vi "add scan PZT at temp.vi"(10 "字符串":string) -> (1 "ok or cancel":bool, 2 "连接的字符串":string)   [LabVIEW 2019, in "nematic.lvlib"]
uses:
  nematic.lvlib
panel:
  out "数组 2":i32[](array[numeric])
  out "布尔":bool
  in  "最大电压":dbl=148.0
  in  "最小电压":dbl=-48.0
  in  "ok 2":bool
  in  "cancel":bool
  in  "ok":bool
  in  "零电压":dbl
  in  "间隔":dbl=4.0
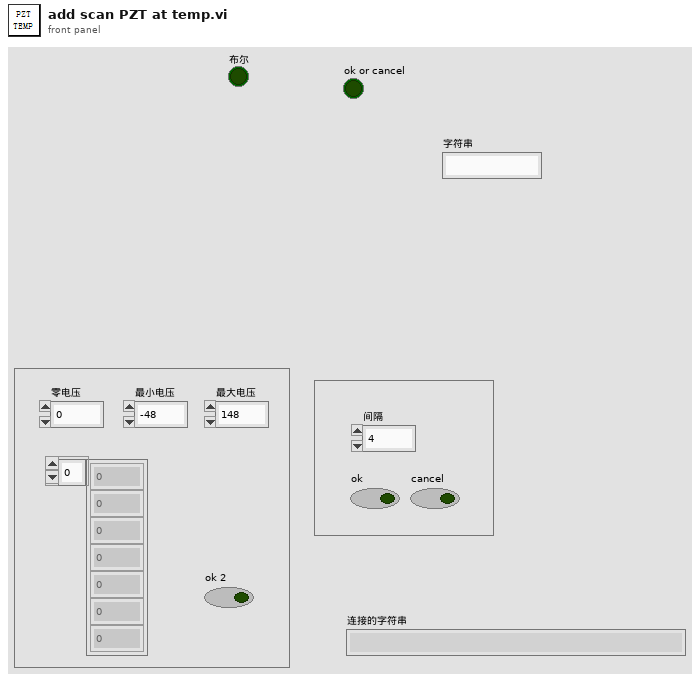
[diagram p1: front panel]
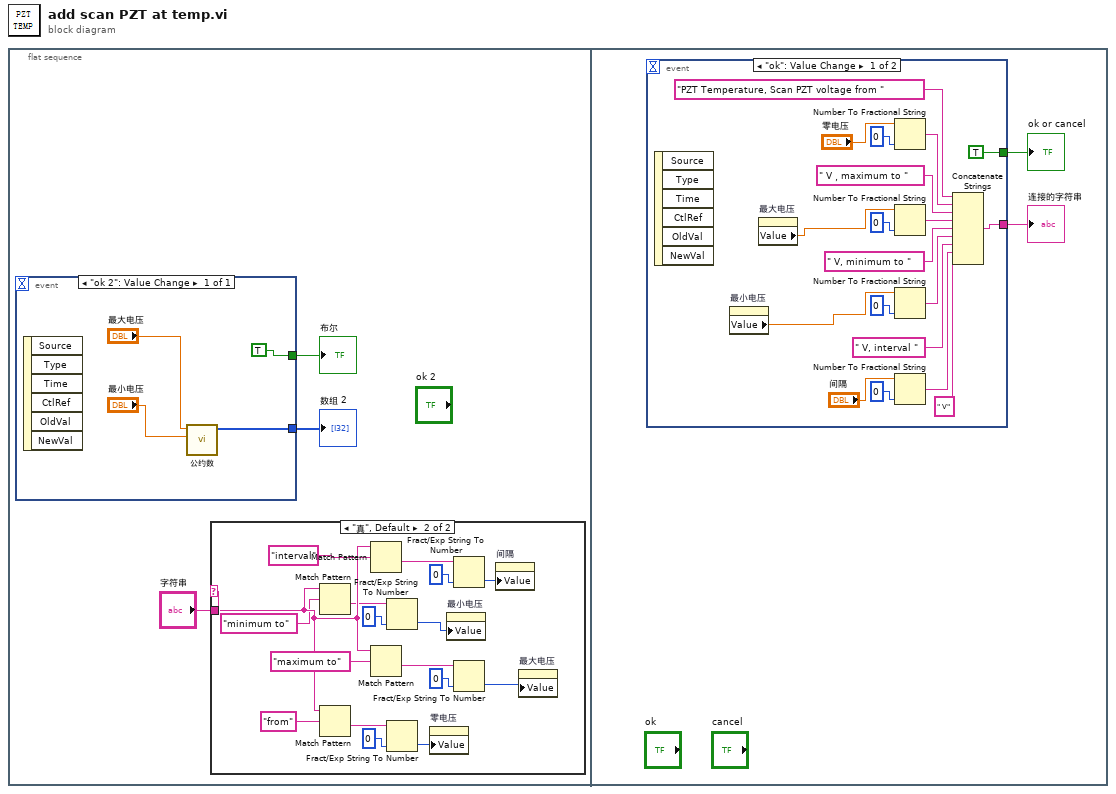
[diagram p0: block diagram]
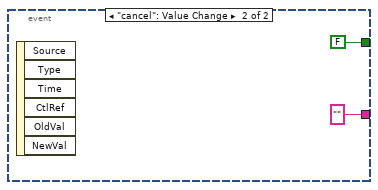
[diagram p3: hidden frame]
diagram:
  n1 = flat-sequence {
    frame #0 {
      n2 = event shown="[0] \"ok 2\": Value Change" {
        selector: _ -> [_]
        dyn-events: _ -> [_]
        timeout: _ -> [_]
        tunnel: [TRUE] -> w3
        tunnel: [w21] -> w2
        event "ok 2": Value Change {
          n3 = event-data() -> ()  [unwired: 1 in, 6 out]
          n4 = call "公约数.vi"("数值 2"="最小电压", "数值"="最大电压") -> ("数组"=w21:i32[])  [unwired: 8 in, 1 out]
        }
      }
      "布尔" <- w3
      "数组 2" <- w2
      n5 = case shown="\"真\", Default" "字符串" {
        tunnel: "字符串" -> [_ w16]
        frame "" {
        }
        frame "真", Default {
          n6 = Match Pattern(string=w16, regular expression="minimum to" ("正则表达式")) -> (after substring=w9:string)  [unwired: 1 in, 3 out]
          n7 = Match Pattern(string=w16, regular expression="from" ("正则表达式")) -> (after substring=w18:string)  [unwired: 1 in, 3 out]
          n8 = Match Pattern(string=w16, regular expression="interval" ("正则表达式")) -> (after substring=w8:string)  [unwired: 1 in, 3 out]
          n9 = Match Pattern(string=w16, regular expression="maximum to" ("正则表达式")) -> (after substring=w10:string)  [unwired: 1 in, 3 out]
          n10 = Fract/Exp String To Number(string=w9, default (0 dbl)=0) -> (number=w5:i32)  [unwired: 2 in, 1 out]
          n11 = Fract/Exp String To Number(string=w18, default (0 dbl)=0) -> (number=w7:i32)  [unwired: 2 in, 1 out]
          n12 = property on="零电压" class="DigNum (strict)"("Value"=w7) -> ()  [unwired: 2 in, 2 out]
          n13 = property on="最小电压" class="DigNum (strict)"("Value"=w5) -> ()  [unwired: 2 in, 2 out]
          n14 = Fract/Exp String To Number(string=w8, default (0 dbl)=0) -> (number=w6:i32)  [unwired: 2 in, 1 out]
          n15 = Fract/Exp String To Number(string=w10, default (0 dbl)=0) -> (number=w4:i32)  [unwired: 2 in, 1 out]
          n16 = property on="间隔" class="DigNum (strict)"("Value"=w6) -> ()  [unwired: 2 in, 2 out]
          n17 = property on="最大电压" class="DigNum (strict)"("Value"=w4) -> ()  [unwired: 2 in, 2 out]
        }
      }
    }
    frame #1 {
      n18 = event shown="[0] \"ok\": Value Change" {
        selector: _ -> [_ _]
        dyn-events: _ -> [_ _]
        timeout: _ -> [_ _]
        tunnel: [TRUE FALSE] -> w25
        tunnel: [w37 "" ("分隔符")] -> w26
        event "ok": Value Change {
          n19 = event-data() -> ()  [unwired: 1 in, 6 out]
          n20 = property on="最小电压" class="DigNum (strict)"() -> ("Value"=w27:dbl)  [unwired: 2 in, 2 out]
          n21 = property on="最大电压" class="DigNum (strict)"() -> ("Value"=w28:dbl)  [unwired: 2 in, 2 out]
          n22 = Number To Fractional String(number="零电压", precision (6)=i16 0 ("精度(6)")) -> (F-format string=w43:string)  [unwired: 2 in]
          n23 = Number To Fractional String(number=w28, precision (6)=i16 0 ("精度(6)")) -> (F-format string=w39:string)  [unwired: 2 in]
          n24 = Number To Fractional String(number=w27, precision (6)=i16 0 ("精度(6)")) -> (F-format string=w34:string)  [unwired: 2 in]
          n25 = Number To Fractional String(number="间隔", precision (6)=i16 0 ("精度(6)")) -> (F-format string=w30:string)  [unwired: 2 in]
          n26 = Concatenate Strings("PZT Temperature, Scan PZT voltage from " ("字符串"), w43, " V，maximum to " ("字符串"), w39, " V, minimum to " ("字符串"), w34, " V, interval " ("字符串"), w30, " V" ("string")) -> (w37:string)
        }
        event "cancel": Value Change {
          n27 = event-data() -> ()  [unwired: 1 in, 6 out]
        }
      }
      "ok or cancel" <- w25
      "连接的字符串" <- w26
    }
  }
